vi "TCP Open (port).vi"(6 "local port (0)":u16, 8 "error in (no error)":errorcluster, 9 "timeout ms (60000)":i32=60000, 10 "remote port or service name":u16, 11 "address":string) -> (0 "error out":errorcluster, 3 "TCP out":refnum<class "TCP.lvclass">)   [LabVIEW 2013, in "TCP.lvclass"]
doc: "Opens a TCP network connection"
uses:
  TCP.lvclass
  TCP.lvclass/TCP.ctl
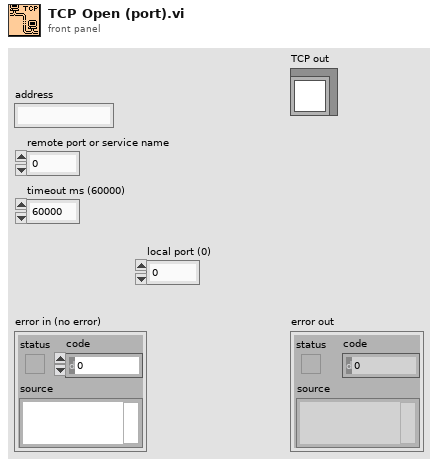
[diagram p1: front panel]
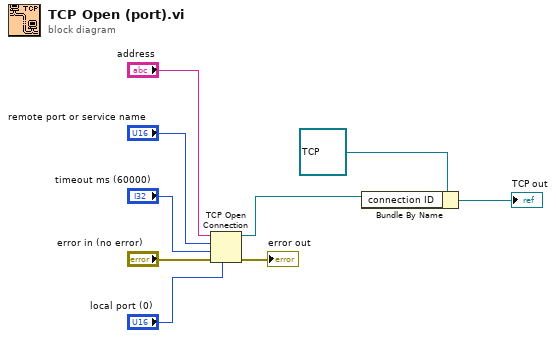
[diagram p0: block diagram]
diagram:
  n1 = TCP Open Connection(address="address", remote port or service name="remote port or service name", timeout ms (60000)="timeout ms (60000)", local port="local port (0)", error in (no error)="error in (no error)") -> (connection ID=w3:refnum<k5>, error out=→"error out":errorcluster)
  n2 = Bundle By Name(cluster=refnum<class "TCP.lvclass"> refnum ("TCP out"), "connection ID"=w3) -> (→"TCP out":refnum<class "TCP.lvclass">)
